vi "ZDataVIS_Configure_Linecuts.vi"(5 "X Offset+Mult":cluster{"Offset X Low":dbl, "X Step":dbl}, 6 "XYZ Variable Selection":T1, 7 "Scan Name":string[](array[string]), 8 "error in (no error)":errorcluster, 9 "swap x and y?":bool=TRUE, 10 "Y line cut":refnum<vi>, 11 "X line cut":refnum<vi>) -> (0 "error out":errorcluster)   [LabVIEW 2016]
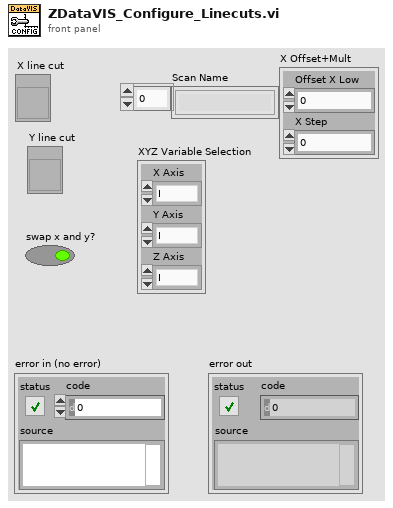
[diagram p1: front panel]
types:
  T1 = cluster{"X Axis":enum16{"I", "Vsd", "V4T", "dI/dV 2T", "dV/dI 2T", "dV/dI 4T", "dI/dV 4T"}, "Y Axis":enum16{"I", "Vsd", "V4T", "dI/dV 2T", "dV/dI 2T", "dV/dI 4T", "dI/dV 4T"}, "Z Axis":enum16{"I", "Vsd", "V4T", "dI/dV 2T", "dV/dI 2T", "dV/dI 4T", "dI/dV 4T"}}
  T2 = enum16{"I", "Vsd", "V4T", "dI/dV 2T", "dV/dI 2T", "dV/dI 4T", "dI/dV 4T"}
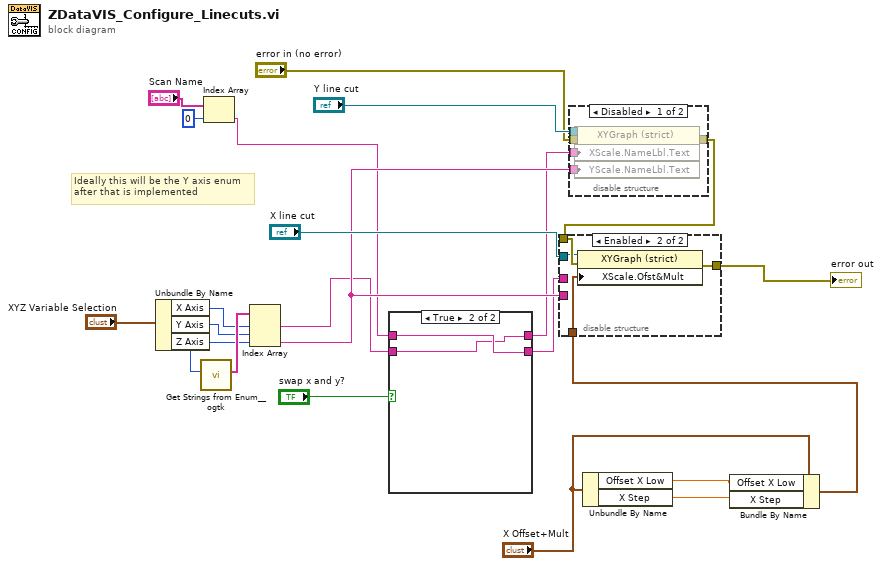
[diagram p0: block diagram]
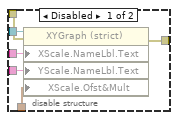
[diagram p2: hidden frame]
diagram:
  # "Ideally this will be the Y axis enum\nafter that is implemented"
  n1 = Unbundle By Name("XYZ Variable Selection") -> ("X Axis"=w20:T2, "Y Axis"=w19:T2, "Z Axis"=w18:T2)
  n2 = call <userlib>:"Get Strings from Enum__ogtk.vi"("Enum"=w18) -> ("Enum Strings"=w21:string[])  [unwired: 7 in, 3 out]
  n3 = Index Array(array="Scan Name", index=0) -> (element=w7:string)
  n4 = Index Array(array=w21, index #1=w20, index #2=w19, index #3=w18) -> (element #1=w9:string, element #3=w10:string)  [unwired: 1 out]
  n5 = case shown="True" "swap x and y?" {
    tunnel: w9 -> [w24 w25]
    tunnel: [w24 w26] -> w8
    tunnel: w7 -> [w23 w26]
    tunnel: [w23 w25] -> w6
    frame False {
    }
    frame True {
    }
  }
  n6 = disable-structure shown="Disabled" {
    disable-tunnel: "Y line cut" -> [w31 _]
    disable-tunnel: "error in (no error)" -> [w30 _]
    disable-tunnel: [w29 _] -> w12
    disable-tunnel: w10 -> [w28 _]
    disable-tunnel: w6 -> [w27 _]
    frame Disabled {
      n7 = property class="XYGraph (strict)"(reference=w31, error in=w30, "XScale.NameLbl.Text"=w27, "YScale.NameLbl.Text"=w28) -> (error out=w29:errorcluster)  [unwired: 1 out]
    }
    frame Enabled {
    }
  }
  n8 = Unbundle By Name("X Offset+Mult") -> ("Offset X Low"=w2:dbl, "X Step"=w1:dbl)
  n9 = Bundle By Name(cluster="X Offset+Mult", "Offset X Low"=w2, "X Step"=w1) -> (w3:cluster{"Offset X Low":dbl, "X Step":dbl})
  n10 = disable-structure shown="Enabled" {
    disable-tunnel: "X line cut" -> [w37 w38]
    disable-tunnel: w12 -> [w36 w39]
    disable-tunnel: [w35 w40] -> w11
    disable-tunnel: w10 -> [w34 _]
    disable-tunnel: w8 -> [w33 _]
    disable-tunnel: w3 -> [w32 w41]
    frame Disabled {
      n11 = property class="XYGraph (strict)"(reference=w37, error in=w36, "XScale.NameLbl.Text"=w33, "YScale.NameLbl.Text"=w34, "XScale.Ofst&Mult"=w32) -> (error out=w35:errorcluster)  [unwired: 1 out]
    }
    frame Enabled {
      n12 = property class="XYGraph (strict)"(reference=w38, error in=w39, "XScale.Ofst&Mult"=w41) -> (error out=w40:errorcluster)  [unwired: 1 out]
    }
  }
  "error out" <- w11
